vi "Factorial.vi"(10 "Factorial of Integer N":dbl) -> (2 "N!":dbl format="%.6f")   [LabVIEW 2017]
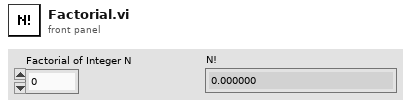
[diagram p1: front panel]
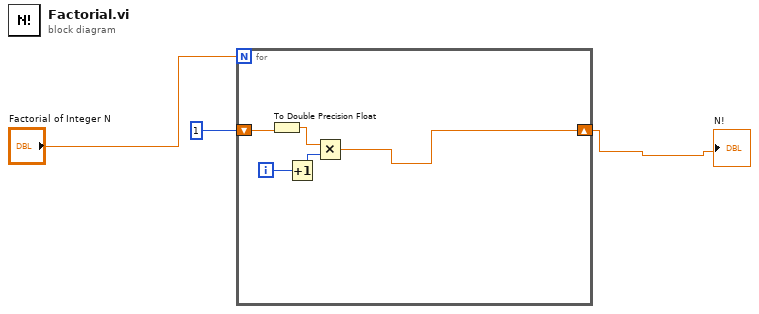
[diagram p0: block diagram]
diagram:
  n1 = for {
    N: "Factorial of Integer N" -> [_]
    shift-right: [w4] -> w1
    shift-left: 1 -> [w6]
    i -> [w8]
    n2 = To Double Precision Float(number=w6) -> (double precision float=w5:dbl)
    n3 = Increment(x=w8) -> (x+1=w7:i32)
    n4 = Multiply(x=w5, y=w7) -> (x*y=w4:dbl)
  }
  "N!" <- w1
